vi "Point_Set_Valid.vi"(6 "Timestamp":timestamp, 8 "Error In":errorcluster, 9 "Valid?":bool, 10 "Tag":string, 11 "Map":T1) -> (0 "Error Out":errorcluster, 3 "Map Out":T1)   [LabVIEW 2017, in "PointValueMap.lvlib"]
doc: "Sets an attribute on a map point that indicates whether the point contains a valid value. You can use this attribute to determine whether to act on the point value or to ignore it. The Point Read VI returns the value of this attribute if you set one."
uses:
  <vilib>/addons/PointValueMap/PointValueMap.lvlib
  <vilib>/addons/PointValueMap/controls/PointMap.ctl
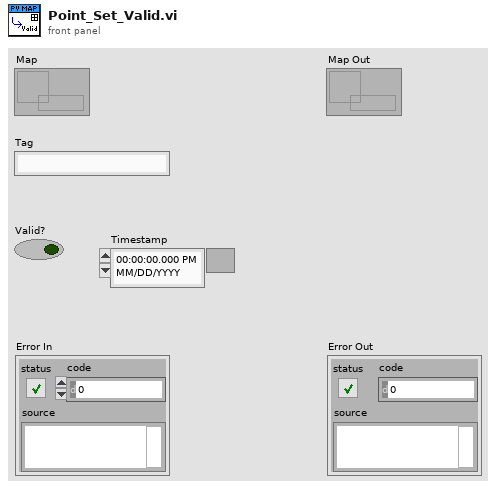
[diagram p1: front panel]
types:
  T1 = typedef "PointValueMap.lvlib/PointMap.ctl" = refnum<data-value>
  T2 = typedef "PointValueMap.lvlib/Point.ctl" = cluster{"Datatype":T3, "Timestamp":timestamp, "Value":variant, "Valid":bool}
  T3 = typedef "PointValueMap.lvlib/DataTypes.ctl" = enum16{"single", "double", "i32", "string", "variant"}
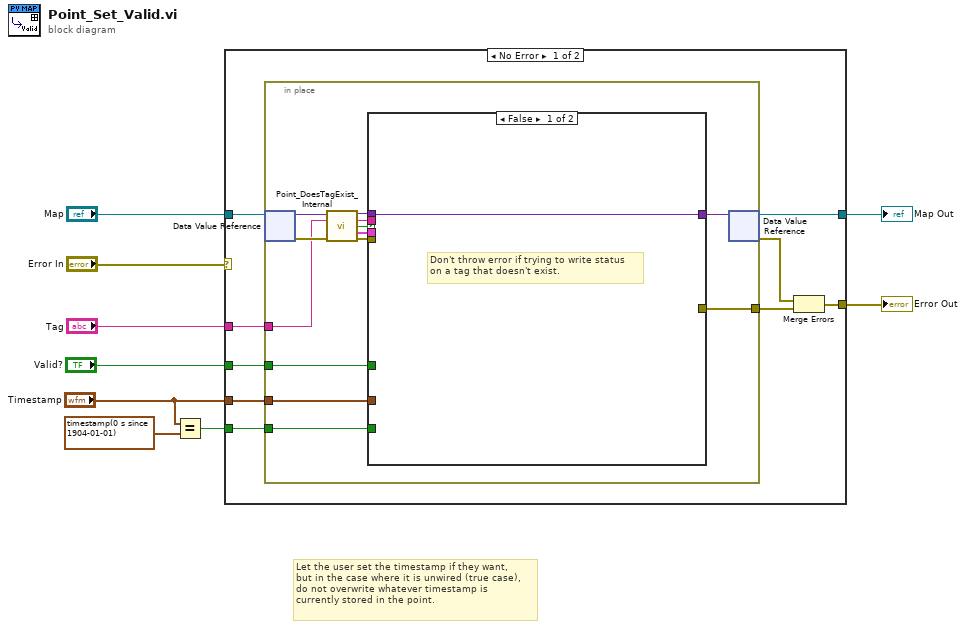
[diagram p0: block diagram]
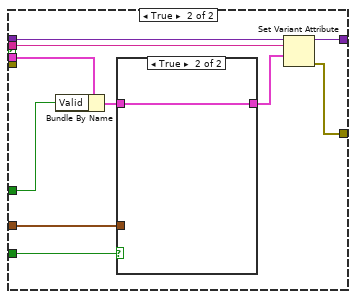
[diagram p2: hidden frame]
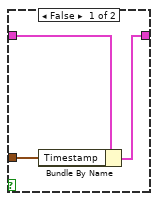
[diagram p3: hidden frame]
diagram:
  # "Let the user set the timestamp if they want,\nbut in the case where it is unwired (true case),\ndo not overwrite whatever timestamp is \ncurrently stored in the point."
  n1 = Equal?(x="Timestamp", y=timestamp(0 s since 1904-01-01) ("Timestamp")) -> (x = y?=w2:bool)
  n2 = case shown="No Error" "Error In" {
    selector: "Error In" -> [_ w48]
    tunnel: "Map" -> [w18 w47]
    tunnel: "Tag" -> [w17 _]
    tunnel: [w14 w48] -> w8
    tunnel: [w13 w47] -> w5
    tunnel: "Valid?" -> [w12 _]
    tunnel: w2 -> [w11 _]
    tunnel: "Timestamp" -> [w10 _]
    frame No Error {
      n3 = in-place {
        in-place-border: w17 -> [w24]
        in-place-border: [w30] -> w15
        in-place-border: w12 -> [w21]
        in-place-border: w11 -> [w20]
        in-place-border: w10 -> [w19]
        n4 = in-place-dvr #1(w18) -> (w29:variant, w27:errorcluster)
        n5 = call <vilib>:"Point_DoesTagExist_Internal.vi"("Map"=w29, "Tag"=w24, "Error In"=w27) -> ("Map Out"=w28:variant, "Tag Out"=w22:string, "Tag Exists"=w25:bool, "Point"=w23:T2, "Error Out"=w26:errorcluster)  [unwired: 7 in, 1 out]
        n6 = case shown="False" w25 {
          tunnel: [w32 w42] -> w31
          tunnel: [_ w41] -> w30
          tunnel: w28 -> [w32 w40]
          tunnel: w26 -> [_ _]
          tunnel: w23 -> [_ w39]
          tunnel: w22 -> [_ w38]
          tunnel: w21 -> [_ w37]
          tunnel: w20 -> [_ w34]
          tunnel: w19 -> [_ w33]
          frame False {
            # "Don't throw error if trying to write status\non a tag that doesn't exist."
          }
          frame True {
            n7 = Bundle By Name(cluster=w39, "Valid"=w37) -> (w35:T2)
            n8 = case shown="True" w34 {
              tunnel: [w44 w46] -> w36
              tunnel: w35 -> [w45 w46]
              tunnel: w33 -> [w43 _]
              frame False {
                n9 = Bundle By Name(cluster=w45, "Timestamp"=w43) -> (w44:T2)
              }
              frame True {
              }
            }
            n10 = Set Variant Attribute(Variant=w40, name=w38, value=w36) -> (Variant out=w42:variant, error out=w41:errorcluster)  [unwired: 1 in, 1 out]
          }
        }
        n11 = in-place-dvr #1(w31) -> (w13:T1, w16:errorcluster)
      }
      n12 = Merge Errors(w16, w15) -> (w14:errorcluster)
    }
    frame Error {
    }
  }
  "Error Out" <- w8
  "Map Out" <- w5
